vi "write_symbols_to_project_item.vi"(8 "error in (no error)":errorcluster, 9 "Updated":map{string, string}(c390), 11 "ProjectItem in":refnum<vi>) -> (0 "error out":errorcluster, 3 "ProjectItem out":refnum<vi>)   [LabVIEW 2019, in "Conditional Disable Build Actions.lvlib"]
uses:
  Conditional Disable Build Actions.lvlib
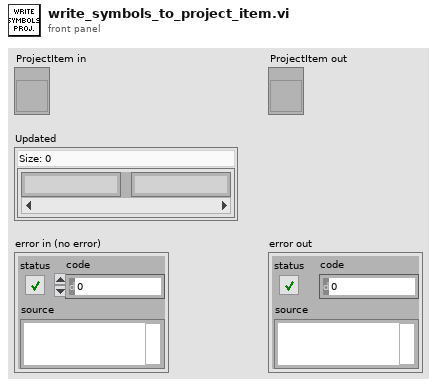
[diagram p1: front panel]
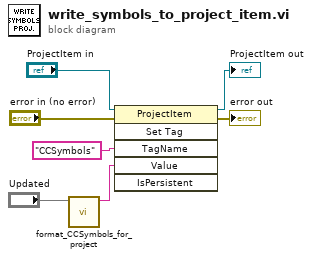
[diagram p0: block diagram]
diagram:
  n1 = call "format_CCSymbols_for_project.vi"("CCSymbols"="Updated") -> ("CCSymbols for project"=w6:string)  [unwired: 10 in]
  n2 = invoke class="ProjectItem" method="Set Tag"(reference="ProjectItem in", error in="error in (no error)", "TagName"="CCSymbols" ("Tag Name"), "Value"=w6) -> (reference out=→"ProjectItem out":refnum<vi>, error out=→"error out":errorcluster)  [unwired: 2 in, 4 out]
